vi "d.vi"(8 "error in (no error)":errorcluster, 9 "d Cmd Properties":T1, 11 "ArrayController in":refnum<class "ArrayController.lvclass">) -> (0 "error out":errorcluster, 3 "ArrayController out":refnum<class "ArrayController.lvclass">)   [LabVIEW 2018, in "ArrayController.lvclass"]
uses:
  ArrayController.lvclass
  Datalog/DatalogSubvis/SearchableTag.ctl
  Sequence/SequenceSubvis/RF Direction.ctl
  Sequence/SequenceSubvis/PolarizationSelect.ctl
  ArrayController.lvclass/ArrayController.ctl
  <vilib>/DAQmx/write.llb/DAQmx Write (Analog 1D DBL NChan 1Samp).vi
  <vilib>/DAQmx/miscellaneous.llb/DAQmx Fill In Error Info.vi
  Datalog/DataLog.lvclass
panel:
  # "Address, T, R, H, V, Phase, Attenuation"
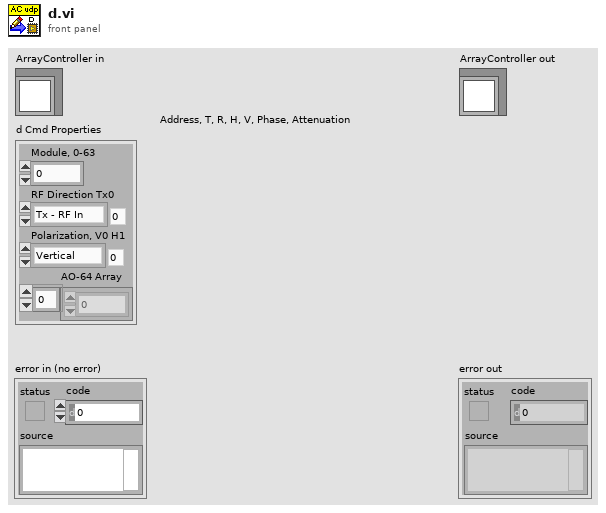
[diagram p1: front panel]
types:
  T1 = typedef "DataLog.lvclass/SearchableTag.ctl" = cluster{"Module, 0-63":i32, "RF Direction Tx0":T2, "Polarization, V0 H1":T3, "AO-64 Array":dbl[]}
  T2 = typedef "RF Direction.ctl" = enum16{"Tx - RF In", "Rx - RF Out"}
  T3 = typedef "PolarizationSelect.ctl" = enum16{"Vertical", "Horizontal"}
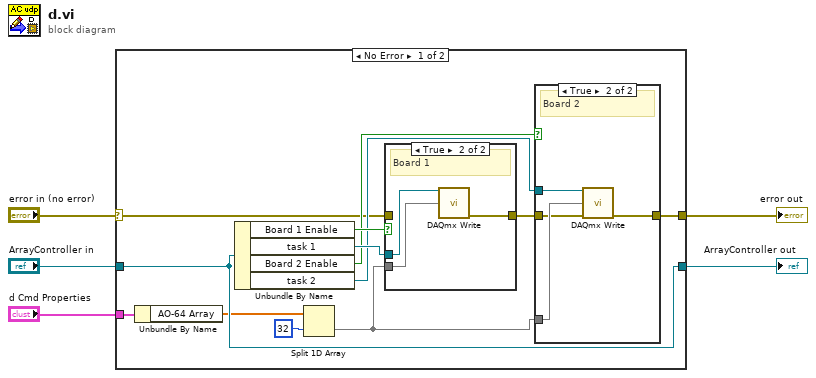
[diagram p0: block diagram]
diagram:
  n1 = case shown="No Error" "error in (no error)" {
    selector: "error in (no error)" -> [w6 w28]
    tunnel: [w7 w28] -> w4
    tunnel: [w17 w27] -> w2
    tunnel: "ArrayController in" -> [w17 w27]
    tunnel: "d Cmd Properties" -> [w15 _]
    frame No Error {
      n2 = Unbundle By Name(w15) -> ("AO-64 Array"=w14:dbl[])
      n3 = Unbundle By Name(w17) -> ("Board 1 Enable"=w12:bool, "task 1"=w16:refnum<k21>, "Board 2 Enable"=w11:bool, "task 2"=w10:refnum<k21>)
      n4 = Split 1D Array(array=w14, index=32) -> (second subarray=w9:dbl[])  [unwired: 1 out]
      n5 = case shown="True" w12 {
        tunnel: w16 -> [_ w26]
        tunnel: w9 -> [_ w25]
        tunnel: [w23 w24] -> w8
        tunnel: w6 -> [w23 _]
        frame False {
        }
        frame True {
          # "Board 1"
          n6 = call-poly <vilib>:"DAQmx Write.vi"("task/channels in"=w26, "data"=w25) -> ("error out"=w24:errorcluster)  [unwired: 11 in, 2 out]
        }
      }
      n7 = case shown="True" w11 {
        tunnel: w10 -> [_ w22]
        tunnel: w9 -> [_ w21]
        tunnel: w8 -> [w18 w20]
        tunnel: [w18 w19] -> w7
        frame False {
        }
        frame True {
          # "Board 2"
          n8 = call-poly <vilib>:"DAQmx Write.vi"("task/channels in"=w22, "data"=w21, "error in"=w20) -> ("error out"=w19:errorcluster)  [unwired: 10 in, 2 out]
        }
      }
    }
    frame Error {
    }
  }
  "error out" <- w4
  "ArrayController out" <- w2
